vi "Adjust Text to Fit Rectangle.vi"(0 "VI Name":string, 5 "Number of Rows":i32, 7 "Text settings":T1 {"Alignment" items=["left", "center", "right"]}) -> (4 "Text out":T4)   [LabVIEW 2020, in "Text-Based VI Icon.lvlib"]
uses:
  <vilib>/LabVIEW Icon API/Set Text Icon/Text-Based VI Icon.lvlib
  <vilib>/LabVIEW Icon API/API_Text.ctl
  <vilib>/LabVIEW Icon API/LabVIEW Icon API.lvlib
  <vilib>/LabVIEW Icon API/lv_icon/Controls/Alignment.ctl
  <vilib>/LabVIEW Icon API/API_Text Colors.ctl
  <vilib>/LabVIEW Icon API/API_Test Settings.ctl
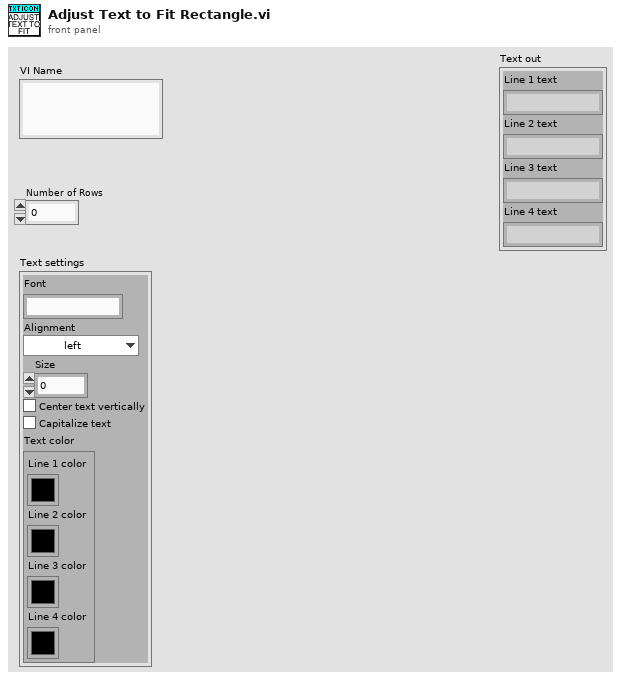
[diagram p1: front panel]
types:
  T1 = typedef "LabVIEW Icon API.lvlib/API_Test Settings.ctl" = cluster{"Font":string, "Alignment":T2, "Size":u8, "Center text":bool, "Capitalize text":bool, "Text color":T3}
  T2 = typedef "Alignment.ctl" = u16
  T3 = typedef "LabVIEW Icon API.lvlib/API_Text Colors.ctl" = cluster{"Line 1 color":u32, "Line 2 color":u32, "Line 3 color":u32, "Line 4 color":u32}
  T4 = typedef "LabVIEW Icon API.lvlib/API_Text.ctl" = cluster{"Line 1 text":string, "Line 2 text":string, "Line 3 text":string, "Line 4 text":string}
  T5 = cluster{"Font Name:":string, "Size":i16, "Strikeout?":bool, "Italic?":bool, "Underline?":bool, "Outline?":bool, "Shadow?":bool, "Bold?":bool}
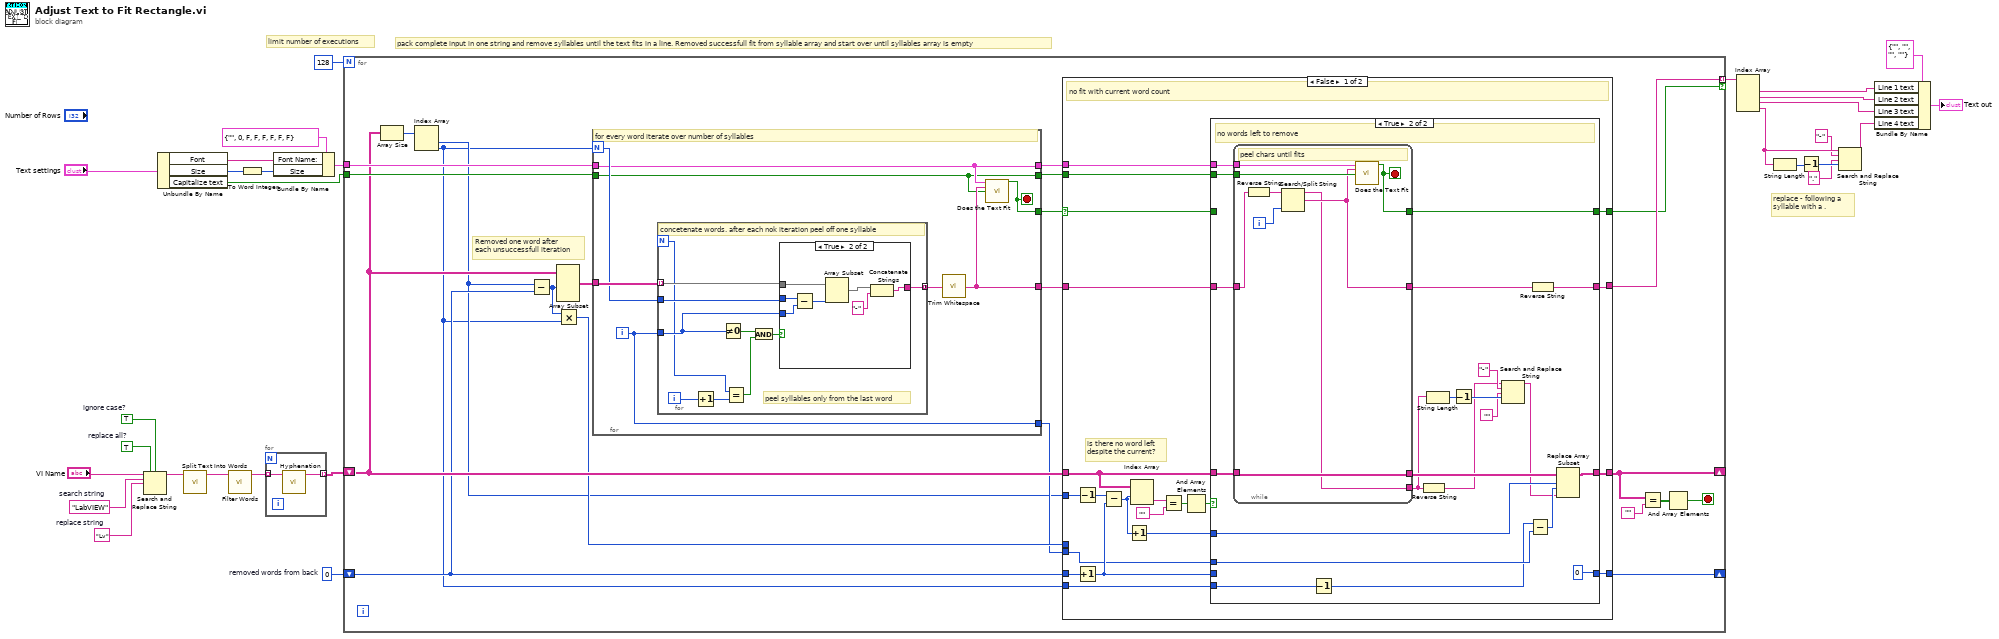
[diagram p0: block diagram]
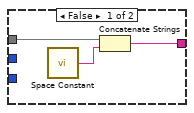
[diagram p2: hidden frame]
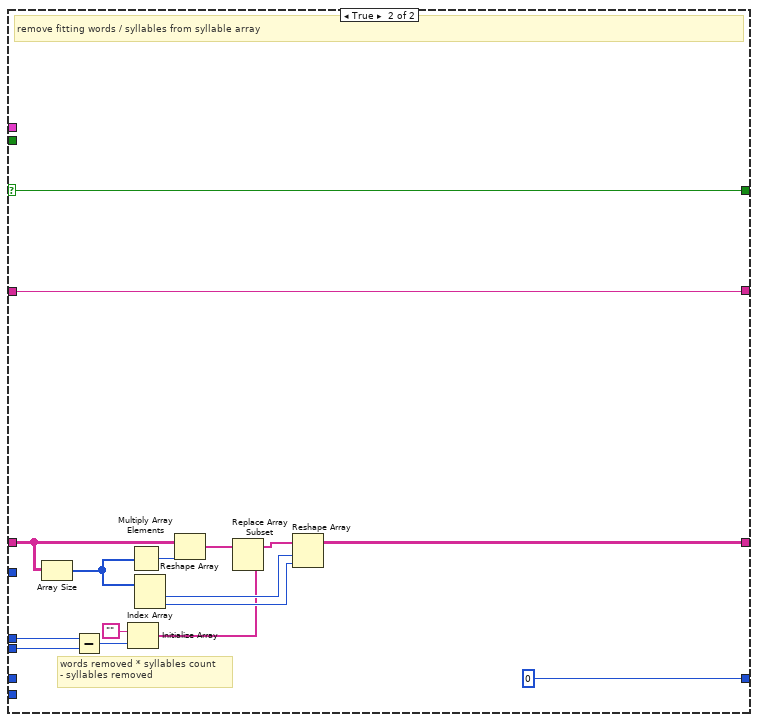
[diagram p4: hidden frame]
diagram:
  w10 = 0  # removed words from back
  w14 = TRUE  # ignore case?
  w15 = TRUE  # replace all?
  w16 = "Lv"  # replace string
  w17 = "LabVIEW"  # search string
  # "pack complete input in one string and remove syllables until the text fits in a line. Removed successfull fit from syllable array and start over until syllables array is empty"
  # "replace - following a\nsyllable with a ."
  # "limit number of executions"
  n1 = Search and Replace String(replace all?=w15, case sensitive?=w14, input string="VI Name", search string=w17, replace string=w16) -> (result string=w12:string)  [unwired: 3 in, 3 out]
  n2 = Unbundle By Name("Text settings") -> ("Font"=w23:string, "Size"=w22:u8, "Capitalize text"=w19:bool)
  n3 = call <vilib>:"Split Text Into Words.vi"("VI Name"=w12) -> ("Array"=w18:string[])  [unwired: 10 in]
  n4 = call <vilib>:"Filter Words.vi"("Array in"=w18) -> ("Array out"=w11:string[])  [unwired: 10 in]
  n5 = To Word Integer(number=w22) -> (16bit integer=w20:i16)
  n6 = for {
    tunnel: w11 -> [w32] mode=indexing
    tunnel: [w31] -> w9 mode=indexing
    n7 = call "Hyphenation.vi"("Word"=w32) -> ("Hyphenated"=w31:string[])  [unwired: 9 in, 1 out]
  }
  n8 = Bundle By Name(cluster=T5 {"Font Name:"="", "Size"=0, "Strikeout?"=FALSE, "Italic?"=FALSE, "Underline?"=FALSE, "Outline?"=FALSE, "Shadow?"=FALSE, "Bold?"=FALSE} ("[user-specified font]"), "Font Name:"=w23, "Size"=w20) -> (w2:T5)
  n9 = for {
    N: 128 -> [_]
    tunnel: [w37] -> w26 mode=indexing if=w34
    tunnel: w2 -> [w53]
    tunnel: w19 -> [w52]
    shift-right: [w50] -> _
    shift-left: w9 -> [w51]
    shift-right: [w43] -> _
    shift-left: w10 -> [w40]
    stop <- w41 stop-if-true
    # "Removed one word after\neach unsuccessfull iteration"
    n10 = Array Size(array=w51) -> (size(s)=w54:i32[])
    n11 = Index Array(array=w54) -> (element #1=w39:i32, element #2=w33:i32)  [unwired: 2 in]
    n12 = Subtract(x=w39, y=w40) -> (x-y=w46:i32)
    n13 = Array Subset(array=w51, length (row)=w46) -> (w47:string[][])  [unwired: 3 in]
    n14 = Multiply(x=w46, y=w33) -> (x*y=w45:i32)
    n15 = for {
      N: w33 -> [w58]
      tunnel: [w60] -> w38
      tunnel: w47 -> [w62]
      tunnel: w53 -> [w56]
      tunnel: w52 -> [w55]
      tunnel: [w59] -> w42
      tunnel: [w57] -> w44
      tunnel: [w56] -> w36
      tunnel: [w55] -> w35
      i -> [w57]
      stop <- w59 stop-if-true
      # "for every word iterate over number of syllables"
      n16 = for {
        N -> [w66]
        tunnel: [w72] -> w61 mode=concatenating
        tunnel: w58 -> [w71]
        tunnel: w57 -> [w70]
        tunnel: w62 -> [w69] mode=indexing
        i -> [w64]
        # "peel syllables only from the last word"
        # "concetenate words. after each nok iteration peel off one syllable"
        n17 = Increment(x=w64) -> (x+1=w67:i32)
        n18 = Not Equal To 0?(x=w70) -> (x != 0?=w63:bool)
        n19 = Equal?(x=w66, y=w67) -> (x = y?=w65:bool)
        n20 = And(x=w63, y=w65) -> (x .and. y?=w68:bool)
        n21 = case shown="True" w68 {
          tunnel: [w75 w82] -> w72
          tunnel: w69 -> [w74 w80]
          tunnel: w70 -> [_ w79]
          tunnel: w71 -> [_ w78]
          frame False {
            n22 = call <vilib>:"Space Constant.vi"() -> ("String"=w73:string)
            n23 = Concatenate Strings(w74, w73) -> (w75:string)
          }
          frame True {
            n24 = Subtract(x=w78, y=w79) -> (x-y=w76:i32)
            n25 = Array Subset(array=w80, length=w76) -> (w81:string[])  [unwired: 1 in]
            n26 = Concatenate Strings(w81, "-") -> (w82:string)
          }
        }
      }
      n27 = call <vilib>:"Trim Whitespace.vi"("string"=w61) -> ("trimmed string"=w60:string)  [unwired: 1 in]
      n28 = call <vilib>:"Does the Text Fit.vi"("user-specified font"=w56, "token string"=w60, "Capitalize Text"=w55) -> ("Text Fits"=w59:bool)  [unwired: 12 in]
    }
    n29 = case shown="False" w42 {
      selector: w42 -> [w92 w139]
      tunnel: w51 -> [w97 w154]
      tunnel: [w99 w147] -> w50
      tunnel: w45 -> [_ w148]
      tunnel: w44 -> [w88 w149]
      tunnel: w40 -> [w103 _]
      tunnel: [w95 0] -> w43
      tunnel: w39 -> [w85 _]
      tunnel: w38 -> [w101 w140]
      tunnel: [w100 w140] -> w37
      tunnel: w36 -> [w102 _]
      tunnel: w35 -> [w98 _]
      tunnel: [w91 w139] -> w34
      tunnel: w33 -> [w89 _]
      frame False {
        # "is there no word left\ndespite the current?"
        # "no fit with current word count"
        n30 = Increment(x=w103) -> (x+1=w96:i32)
        n31 = Decrement(x=w85) -> (x-1=w90:i32)
        n32 = Subtract(x=w90, y=w96) -> (x-y=w84:i32)
        n33 = Increment(x=w84) -> (x+1=w83:i32)
        n34 = Index Array(array=w97, index (row)=w84) -> (element=w87:string[])  [unwired: 1 in]
        n35 = Equal?(x=w87, y="") -> (x = y?=w93:bool[])
        n36 = And Array Elements(Boolean array=w93) -> (logical AND=w86:bool)
        n37 = case shown="True" w86 {
          tunnel: w102 -> [_ w129]
          tunnel: w101 -> [w107 w128]
          tunnel: [w107 w115] -> w100
          tunnel: w97 -> [w106 w120]
          tunnel: [w106 w122] -> w99
          tunnel: w98 -> [_ w126]
          tunnel: w96 -> [w105 _]
          tunnel: [w105 0] -> w95
          tunnel: w92 -> [w104 _]
          tunnel: [w104 w124] -> w91
          tunnel: w83 -> [_ w121]
          tunnel: w89 -> [_ w119]
          tunnel: w88 -> [_ w118]
          frame False {
            # "remove a word for next fit check"
          }
          frame True {
            # "no words left to remove"
            n38 = while {
              tunnel: w129 -> [w138]
              tunnel: w128 -> [w137]
              tunnel: [w133] -> w127
              tunnel: w120 -> [w131]
              tunnel: w126 -> [w134]
              tunnel: [w130] -> w109
              tunnel: [w132] -> w124
              tunnel: [w131] -> w123
              i -> [w135]
              stop <- w132 stop-if-true
              # "peel chars until fits"
              n39 = Reverse String(1:w137) -> (0:w136:string)
              n40 = Search/Split String(string=w136, offset (0)=w135) -> (substring before match=w130:string, match + rest of string=w133:string)  [unwired: 1 in, 1 out]
              n41 = call <vilib>:"Does the Text Fit.vi"("user-specified font"=w138, "token string"=w133, "Capitalize Text"=w134) -> ("Text Fits"=w132:bool)  [unwired: 12 in]
            }
            n42 = Decrement(x=w119) -> (x-1=w116:i32)
            n43 = Reverse String(1:w109) -> (0:w110:string)
            n44 = String Length(string=w109) -> (length=w113:i32)
            n45 = Decrement(x=w113) -> (x-1=w114:i32)
            n46 = Search and Replace String(input string=w110, search string="-", replace string="" ("replace string (\"\")"), offset=w114) -> (result string=w108:string)  [unwired: 4 in, 3 out]
            n47 = Subtract(x=w116, y=w118) -> (x-y=w117:i32)
            n48 = Reverse String(1:w127) -> (0:w115:string)
            n49 = Replace Array Subset(array=w123, new element=w108, index (row)=w121, index (col)=w117) -> (w122:string[][])
          }
        }
      }
      frame True {
        # "words removed * syllables count\n- syllables removed"
        # "remove fitting words / syllables from syllable array"
        n50 = Array Size(array=w154) -> (size(s)=w153:i32[])
        n51 = Subtract(x=w148, y=w149) -> (x-y=w144:i32)
        n52 = Initialize Array("", w144) -> (w142:string[])
        n53 = Multiply Array Elements(1:w153) -> (0:w150:i32)
        n54 = Index Array(array=w153) -> (element #1=w146:i32, element #2=w145:i32)  [unwired: 2 in]
        n55 = Reshape Array(w154, w150) -> (w152:string[])
        n56 = Replace Array Subset(array=w152, new element=w142) -> (w151:string[])  [unwired: 1 in]
        n57 = Reshape Array(w151, w146, w145) -> (w147:string[][])
      }
    }
    n58 = Equal?(x=w50, y="") -> (x = y?=w48:bool[][])
    n59 = And Array Elements(Boolean array=w48) -> (logical AND=w41:bool)
  }
  n60 = Index Array(array=w26) -> (element #1=w27:string, element #2=w28:string, element #3=w29:string, element #4=w6:string)  [unwired: 4 in]
  n61 = String Length(string=w6) -> (length=w8:i32)
  n62 = Decrement(x=w8) -> (x-1=w7:i32)
  n63 = Search and Replace String(input string=w6, search string="-", replace string="." ("replace string (\"\")"), offset=w7) -> (result string=w3:string)  [unwired: 4 in, 3 out]
  n64 = Bundle By Name(cluster=T4 {"Line 1 text"="", "Line 2 text"="", "Line 3 text"="", "Line 4 text"=""} ("Text out"), "Line 1 text"=w27, "Line 2 text"=w28, "Line 3 text"=w29, "Line 4 text"=w3) -> (→"Text out":T4)
